vi "Global Constant.vi"() -> ()   [LabVIEW 2019]
panel:
  out "SP_GO_UP":bool
  in  "SP":dbl
  in  "Ziro Level [MPa]":dbl=0.5
  in  "delta P max [MPa]":dbl=25.0
  in  "Breakaway steps [V]":u32=10
  in  "Breakaway voltage [V]":dbl=3.0
  in  "Back Pressure Threshold [MPa]":dbl=1.2
  in  "Back Pressure Range Max [MPa]":dbl=0.8
  in  "Back Pressure Range Min [MPa]":dbl=0.3
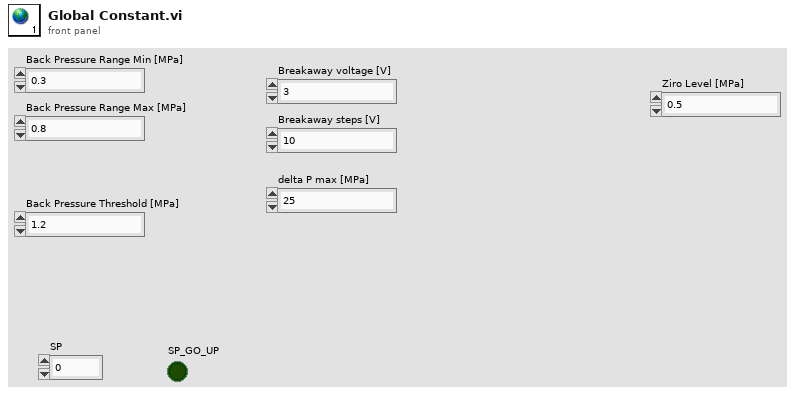
[diagram p1: front panel]
diagram:
